vi "Untitled 7.vi"() -> ()   [LabVIEW 2017]
panel:
  out "find list":string[](array[string])
  out "error out":errorcluster
  out "return count":u32
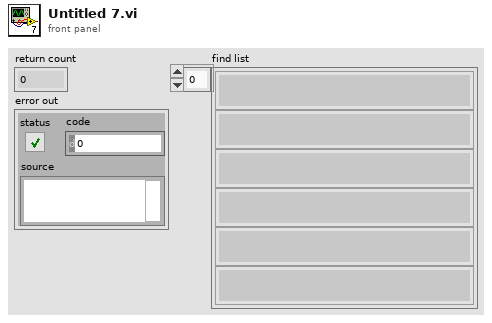
[diagram p1: front panel]
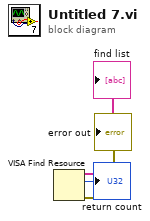
[diagram p0: block diagram]
diagram:
  n1 = VISA Find Resource() -> (0:→"error out":errorcluster, 2:→"return count":u32, 3:→"find list":string[])  [unwired: 3 in]
